vi "RSNRPZ Set Burst Drop-Out Tolerance.vi"(8 "error in (no error)":errorcluster, 9 "Drop-out Tolerance (100.0e-6 s)":dbl=0.0001 format="%.2p", 10 "Channel (1)":i32=1, 11 "VISA session":refnum<visa-resource-name> caption="VISA resource name") -> (0 "error out":errorcluster, 3 "dup VISA session":refnum<visa-resource-name> caption="VISA resource name")   [LabVIEW 2010]
doc: "The end of a burst (power pulse) is recognized when the signal level drops below the trigger level. Especially with modulated signals, this may also happen for a short time within a burst. To prevent the supposed end of the burst is from being recognized too early or incorrectly at these positions, a time interval can be defined via using this VI (drop-out tolerance parameter) in which the pulse end is only recognized if the signal level no longer exceeds the trigger level.\n\nNote:\n\n1) This VI is not available for NRP-Z51\n\nRemote-control command(s):\nSENS:POW:BURS:DTOL"
uses:
  rsnrpz_32.dll
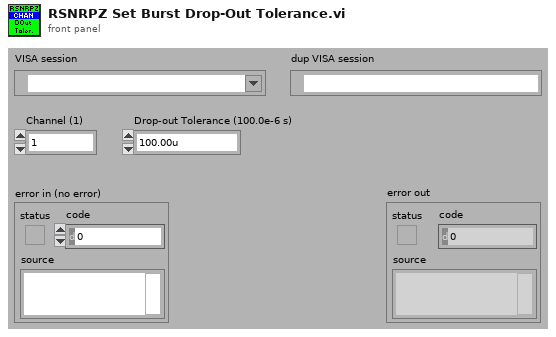
[diagram p1: front panel]
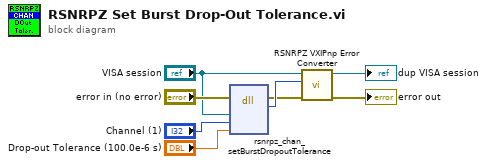
[diagram p0: block diagram]
diagram:
  n1 = dll-call lib="rsnrpz_32.dll" fn="rsnrpz_chan_setBurstDropoutTolerance"(error in="error in (no error)", "VISA Session"="VISA session", "Channel"="Channel (1)", "Drop-out Tolerance"="Drop-out Tolerance (100.0e-6 s)") -> (error out=w5:errorcluster, "Status"=w8:i32)  [unwired: 5 in, 1 out]
  n2 = call <instrlib>:"RSNRPZ VXIPnp Error Converter.vi"("error in"=w5, "VXIPnp error code"=w8, "VISA session"="VISA session") -> ("error out"=→"error out":errorcluster, "dup VISA session"=→"dup VISA session":refnum<visa-resource-name>)  [unwired: 7 in]
